vi "Curvas de uniformidade.vi"(1 "Infos para processamento":T2={"Diâmetro do furo [mm]"=1.4, "Diâmetro da linha média [mm]"=5.0, "IncF"=0.2, "Módulo de elasticidade [GPa]"=207.0, "Módulo de Poisson"=0.3, "Tipo de roseta utilizada"=enum."Tipo A", "Método de análise"=enum."Simplificado 2008", "Pfinal"=0.3, "Parar auto."=TRUE}, 2 "Dados out":T1) -> (0 "Gráficos":cluster{"Array":dbl[], "Array":dbl[]}[](array[cluster]))   [LabVIEW 2016]
uses:
  Controles/Infos para processamento.ctl
  Controles/p,q, t, a e b.ctl
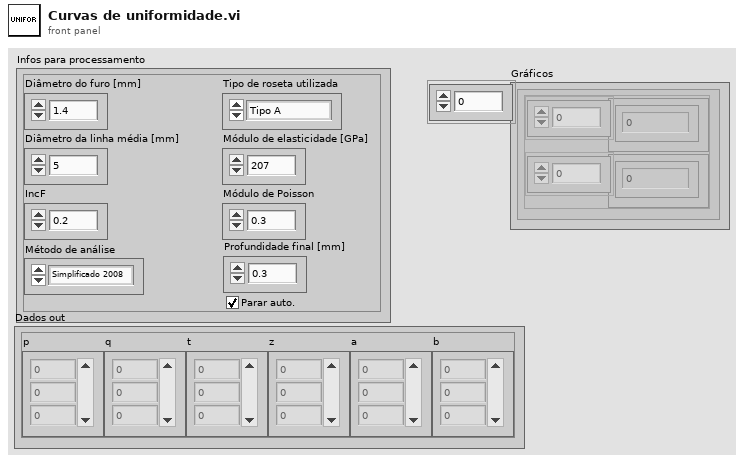
[diagram p1: front panel]
types:
  T1 = typedef "p,q, t, a e b.ctl" = cluster{"p":dbl[], "q":dbl[], "t":dbl[], "z":dbl[], "a":dbl[], "b":dbl[]}
  T2 = typedef "Infos para processamento.ctl" = cluster{"Diâmetro do furo [mm]":dbl, "Diâmetro da linha média [mm]":dbl, "IncF":dbl, "Módulo de elasticidade [GPa]":dbl, "Módulo de Poisson":dbl, "Tipo de roseta utilizada":enum16{"Tipo A", "Tipo B", "Tipo C"}, "Método de análise":enum16{"Não uniforme 2013", "Simplificado 2013", "Simplificado 2008"}, "Pfinal":dbl, "Parar auto.":bool}
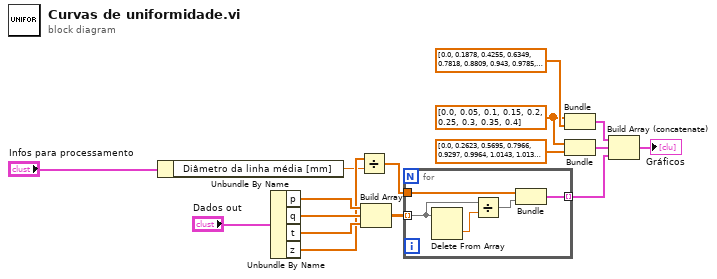
[diagram p0: block diagram]
diagram:
  w6 = dbl[] [0.0, 0.05, 0.1, 0.15, 0.2, 0.25, 0.3, 0.35, 0.4]
  n1 = Unbundle By Name("Infos para processamento") -> ("Diâmetro da linha média [mm]"=w9:dbl)
  n2 = Unbundle By Name("Dados out") -> ("p"=w13:dbl[], "q"=w14:dbl[], "t"=w15:dbl[], "z"=w10:dbl[])
  n3 = Divide(x=w10, y=w9) -> (x/y=w8:dbl[])
  n4 = Build Array(w13, w14, w15) -> (w12:dbl[][])
  n5 = for {
    tunnel: w12 -> [w20] mode=indexing
    tunnel: w8 -> [w19]
    tunnel: [w17] -> w2 mode=indexing
    n6 = Delete From Array(array=w20) -> (deleted portion=w21:dbl)  [unwired: 2 in, 1 out]
    n7 = Divide(x=w20, y=w21) -> (x/y=w18:dbl[])
    n8 = Bundle(w19, w18) -> (w17:cluster{dbl[], dbl[]})  [unwired: 1 in]
  }
  n9 = Bundle(w6, dbl[] [0.0, 0.1878, 0.4255, 0.6349, 0.7818, 0.8809, 0.943, 0.9785, 1.0]) -> (w4:cluster{dbl[], dbl[]})  [unwired: 1 in]
  n10 = Bundle(w6, dbl[] [0.0, 0.2623, 0.5695, 0.7966, 0.9297, 0.9964, 1.0143, 1.0136, 1.0]) -> (w3:cluster{dbl[], dbl[]})  [unwired: 1 in]
  n11 = Build Array (concatenate)(w4, w3, w2) -> (→"Gráficos":cluster{dbl[], dbl[]}[])
